vi "Layout - Parse Layout-VI for Subpanel References.vi"(7 "Layout_VI Ref":refnum<vi>, 8 "error in (no error)":errorcluster, 11 "Subpanel Labels":string[](array[string])) -> (0 "error out":errorcluster, 3 "Subpanel References":refnum<vi>[](array[refnum]))   [LabVIEW 2022 SP3, in "UI Manager.lvlib"]
doc: "Parses the <b>Layout_VI-Ref</b> for subpanels with <b>Subpanel Labels</b> and returns their references.\n\n____\nHAMPEL SOFTWARE ENGINEERING v2.6.0 (2023-12-19 10:54)"
uses:
  UI Manager.lvlib
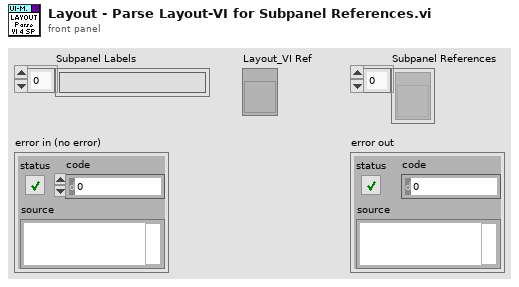
[diagram p1: front panel]
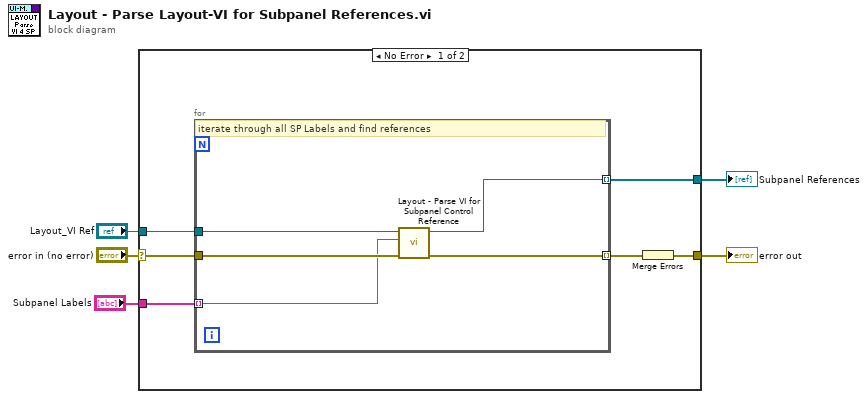
[diagram p0: block diagram]
diagram:
  n1 = case shown="No Error" "error in (no error)" {
    selector: "error in (no error)" -> [w10 w17]
    tunnel: "Layout_VI Ref" -> [w11 _]
    tunnel: "Subpanel Labels" -> [w9 _]
    tunnel: [w7 w17] -> w2
    tunnel: [w6 _] -> w1
    frame No Error {
      n2 = for {
        tunnel: w11 -> [w16]
        tunnel: w10 -> [w15]
        tunnel: w9 -> [w14] mode=indexing
        tunnel: [w13] -> w8 mode=indexing
        tunnel: [w12] -> w6 mode=indexing
        # "iterate through all SP Labels and find references"
        n3 = call "Layout - Parse VI for Subpanel Control Reference.vi"("error in (no error)"=w15, "SubPanel Label"=w14, "VI in"=w16) -> ("error out"=w13:errorcluster, "SubPanel Ref"=w12:refnum<vi>)  [unwired: 7 in]
      }
      n4 = Merge Errors(w8) -> (w7:errorcluster)
    }
    frame Error {
    }
  }
  "error out" <- w2
  "Subpanel References" <- w1
